vi "Seq_array.vi"(5 "Tfail_manual":dbl, 6 "TempSeq in":dbl[][](array[numeric])=[[20.0, 40.0, 1.0, 30.0], [40.0, 50.0, 1.0, 30.0], [50.0, 20.0, 1.0, 30.0], [20.0, 20.0, 0.0, 20.0], [20.0, 20.0, 0.0, 20.0], [20.0, 20.0, 1000.0, 20.0]], 7 "Tmin":dbl, 8 "Tmax":dbl, 9 "Treshold (Tset)":dbl=1.0, 10 "T manual setpoint":dbl=20.0, 11 "Xe":dbl=1.0) -> (2 "TimeParams":dbl[](array[numeric]), 3 "TempParams":dbl[](array[numeric]))   [LabVIEW 2015]
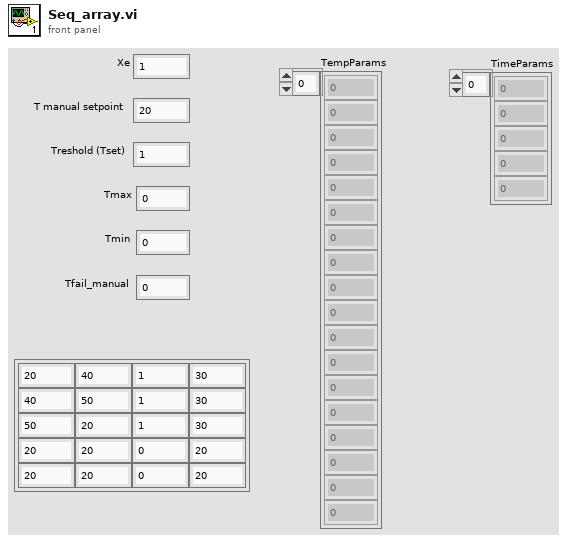
[diagram p1: front panel]
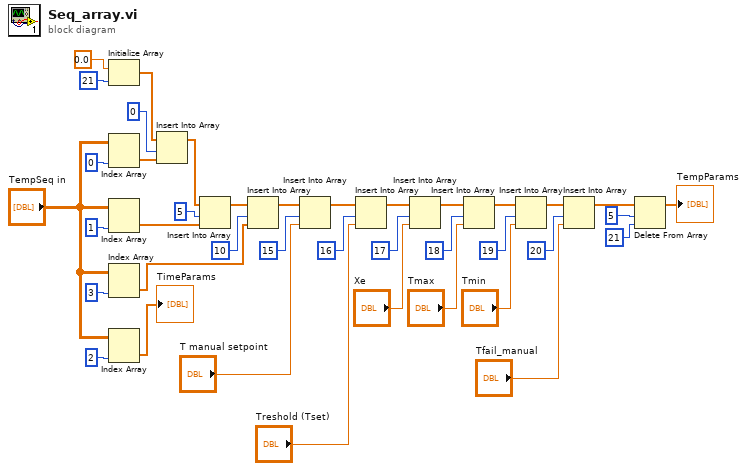
[diagram p0: block diagram]
diagram:
  n1 = Initialize Array(0.0 ("element"), 21 ("dimension size")) -> (w19:dbl[])
  n2 = Index Array(array="TempSeq in", index (col)=0 ("disabled index (col)")) -> (element=w27:dbl[])  [unwired: 1 in]
  n3 = Index Array(array="TempSeq in", index (col)=1 ("disabled index (col)")) -> (element=w31:dbl[])  [unwired: 1 in]
  n4 = Index Array(array="TempSeq in", index (col)=3 ("disabled index (col)")) -> (element=w34:dbl[])  [unwired: 1 in]
  n5 = Index Array(array="TempSeq in", index (col)=2 ("disabled index (col)")) -> (element=→"TimeParams":dbl[])  [unwired: 1 in]
  n6 = Insert Into Array(array=w19, index=0, new element=w27) -> (w30:dbl[])
  n7 = Insert Into Array(array=w30, index=5, new element=w31) -> (w35:dbl[])
  n8 = Insert Into Array(array=w35, index=10, new element=w34) -> (w18:dbl[])
  n9 = Insert Into Array(array=w18, index=15, new element="T manual setpoint") -> (w24:dbl[])
  n10 = Insert Into Array(array=w24, index=16, new element="Treshold (Tset)") -> (w37:dbl[])
  n11 = Insert Into Array(array=w37, index=17, new element="Xe") -> (w10:dbl[])
  n12 = Insert Into Array(array=w10, index=18, new element="Tmax") -> (w9:dbl[])
  n13 = Insert Into Array(array=w9, index=19, new element="Tmin") -> (w8:dbl[])
  n14 = Insert Into Array(array=w8, index=20, new element="Tfail_manual") -> (w1:dbl[])
  n15 = Delete From Array(array=w1, length=5, index=21) -> (array with subset deleted=→"TempParams":dbl[])  [unwired: 1 out]
